vi "Init from Child.vi"(5 "Required Scope(s)":string[](array[string]), 7 "Redirect URL (http://localhost)":string, 8 "error in (no error)":errorcluster, 9 "Token URL":string, 10 "Auth URL":string, 11 "Request in":refnum<class "Request.lvclass">) -> (0 "error out":errorcluster, 3 "Request out":refnum<class "Request.lvclass">)   [LabVIEW 2020]
doc: "Intended to be called by child classes to initialize known values for a given provider, such as the Google authentication URLs."
uses:
  lv-stream/stream/URI/URI.lvclass
  Request.lvclass
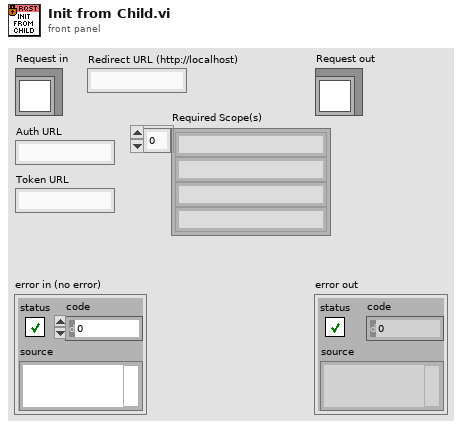
[diagram p1: front panel]
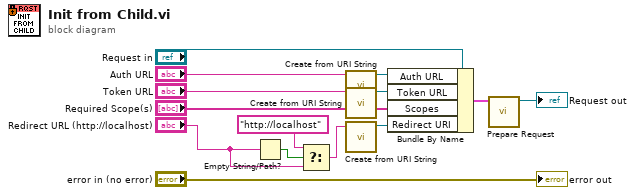
[diagram p0: block diagram]
diagram:
  n1 = Empty String/Path?(string/path="Redirect URL (http://localhost)") -> (empty?=w11:bool)
  n2 = Select(t="http://localhost", s=w11, f="Redirect URL (http://localhost)") -> (s? t:f=w9:string)
  n3 = call "Create from URI String.vi"("URI String"="Auth URL") -> ("URI out"=w13:refnum<class "URI.lvclass">)  [unwired: 9 in, 1 out]
  n4 = call "Create from URI String.vi"("URI String"="Token URL") -> ("URI out"=w12:refnum<class "URI.lvclass">)  [unwired: 9 in, 1 out]
  n5 = call "Create from URI String.vi"("URI String"=w9) -> ("URI out"=w8:refnum<class "URI.lvclass">)  [unwired: 9 in, 1 out]
  n6 = Bundle By Name(cluster="Request in", "Auth URL"=w13, "Token URL"=w12, "Scopes"="Required Scope(s)", "Redirect URI"=w8) -> (w7:cluster{})
  n7 = call "Prepare Request.vi"("Request in"=w7) -> ("Request out"=→"Request out":refnum<class "Request.lvclass">)  [unwired: 10 in]
  "error out" <- "error in (no error)"
